vi "Constructor Basic.vi"(6 "Controller Config":refnum<class "Panel Form Controller Configuration.lvclass">, 8 "error in (no error)":errorcluster, 9 "Panel":refnum<class "Panel.lvclass">, 10 "Panel Form Controller":refnum<class "Panel Form Controller.lvclass">, 11 "Form Model Configuration in":refnum<class "Form Model Configuration.lvclass">) -> (0 "error out":errorcluster, 3 "Form Model Configuration out":refnum<class "Form Model Configuration.lvclass">)   [LabVIEW 2020, in "Form Model Configuration.lvlib" / "Form Model Configuration.lvclass"]
uses:
  Form Model Configuration.lvclass
  <vilib>/MGI/Panel Manager/Panel/Panel/Panel.lvclass
  Form Controller/Panel Form Controller.lvclass
  Controller Configuration/Panel Form Controller Configuration.lvclass
  Form Controller/Panel Form Controller.lvclass/Panel Form Controller.ctl
  Form Model Configuration.lvclass/Form Model Configuration.ctl
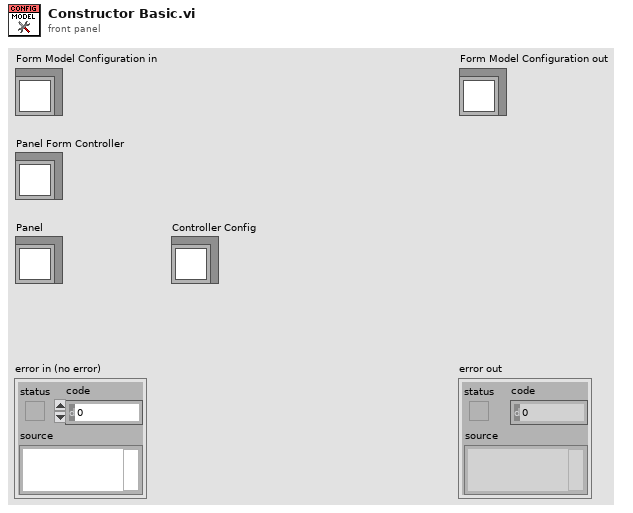
[diagram p1: front panel]
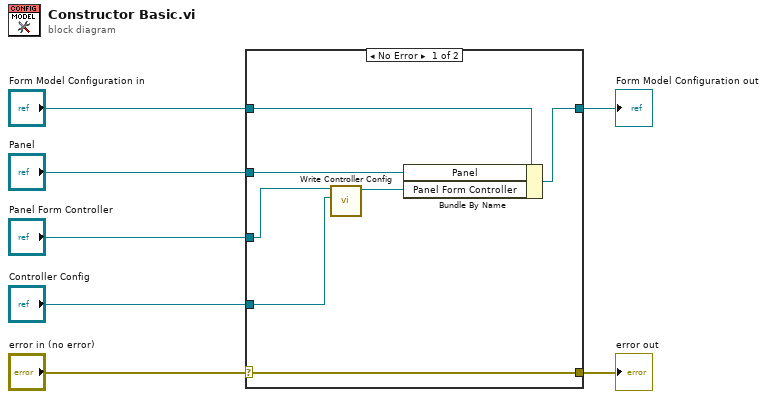
[diagram p0: block diagram]
diagram:
  n1 = case shown="No Error" "error in (no error)" {
    selector: "error in (no error)" -> [w14 w16]
    tunnel: [w14 w16] -> w6
    tunnel: [w13 w15] -> w4
    tunnel: "Form Model Configuration in" -> [w12 w15]
    tunnel: "Panel Form Controller" -> [w10 _]
    tunnel: "Panel" -> [w11 _]
    tunnel: "Controller Config" -> [w9 _]
    frame No Error {
      n2 = call "Write Controller Config.vi"("Controller Config"=w9, "Panel Form Controller in"=w10) -> ("Panel Form Controller out"=w8:refnum<class "Panel Form Controller.lvclass">)  [unwired: 8 in, 1 out]
      n3 = Bundle By Name(cluster=w12, "Panel"=w11, "Panel Form Controller"=w8) -> (w13:refnum<class "Form Model Configuration.lvclass">)
    }
    frame Error {
    }
  }
  "error out" <- w6
  "Form Model Configuration out" <- w4
